vi "n58_manual_status.vi"(8 "error in (no error)":errorcluster, 10 "Research exe":string="\"D:\\River\\DTU_EOL_24\\EXEs\\RESEARCHDOWNLOAD_R22.19.1701\\RESEARCHDOWNLOAD_R22.19.1701_DUT1\\Bin\\ResearchDownload.exe\"") -> (0 "error out":errorcluster, 2 "Status":string)   [LabVIEW 2024]
panel:
  in  "FAIL":bool
  in  "success":bool
  # "N58 FLASH"
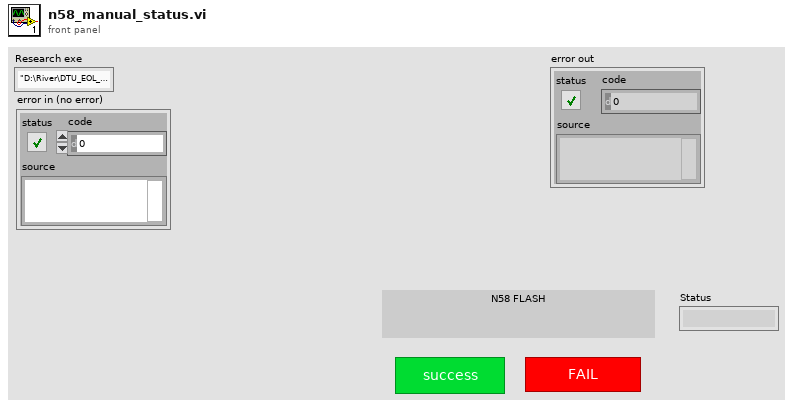
[diagram p1: front panel]
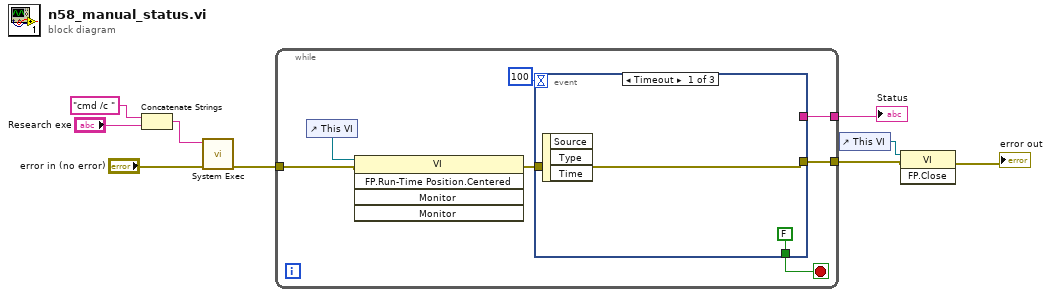
[diagram p0: block diagram]
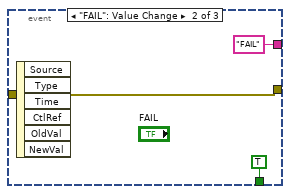
[diagram p2: hidden frame]
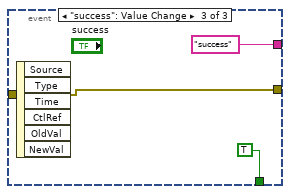
[diagram p3: hidden frame]
diagram:
  n1 = Concatenate Strings("cmd /c ", "Research exe") -> (w7:string)
  n2 = call <vilib>:"System Exec.vi"("error in (no error)"="error in (no error)", "command line"=w7) -> ("error out"=w5:errorcluster)  [unwired: 6 in, 3 out]
  n3 = while {
    tunnel: w5 -> [w11]
    tunnel: [w15] -> w2
    tunnel: [w14] -> w4
    stop <- w13 stop-if-true
    n4 = control-ref of="This VI"() -> (w12:refnum<vi>)
    n5 = invoke class="VI" method="FP.Run-Time Position.Centered"(reference=w12, error in=w11) -> (error out=w10:errorcluster)  [unwired: 3 in, 4 out]
    n6 = event shown="[0] Timeout" {
      selector: _ -> [_ _ _]
      dyn-events: _ -> [_ _ _]
      timeout: 100 -> [_ _ _]
      tunnel: w10 -> [w18 w21 w24]
      tunnel: [w18 w21 w24] -> w15
      tunnel: [_ "FAIL" "success"] -> w14
      tunnel: [FALSE TRUE TRUE] -> w13
      event Timeout {
        n7 = event-data() -> ()  [unwired: 1 in, 3 out]
      }
      event "FAIL": Value Change {
        n8 = event-data() -> ()  [unwired: 1 in, 6 out]
      }
      event "success": Value Change {
        n9 = event-data() -> ()  [unwired: 1 in, 6 out]
      }
    }
  }
  "Status" <- w4
  n10 = control-ref of="This VI"() -> (w3:refnum<vi>)
  n11 = invoke class="VI" method="FP.Close"(reference=w3, error in=w2) -> (error out=→"error out":errorcluster)  [unwired: 1 in, 2 out]
